vi "File Control Time Check.vi"() -> ()   [LabVIEW 2015]
uses:
  <vilib>/Utility/sysdir.llb/System Directory Type.ctl
panel:
  out "x*y":dbl
  out "Data Logging Path":path
  in  "Log no":string="1" caption="No."
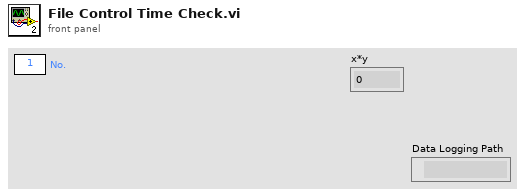
[diagram p1: front panel]
types:
  T1 = enum16{"open", "replace", "create", "open or create", "replace or create", "replace or create with confirmation"}
  T2 = typedef "System Directory Type.ctl" = i32
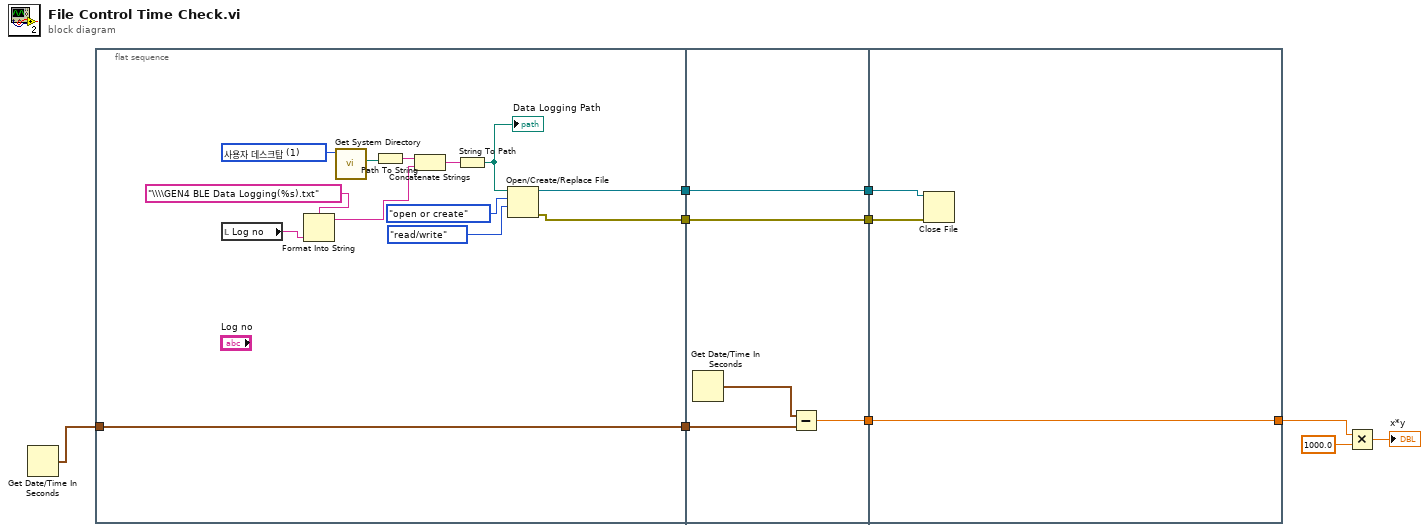
[diagram p0: block diagram]
diagram:
  n1 = Get Date/Time In Seconds() -> (seconds since 1Jan1904=w10:timestamp)
  n2 = flat-sequence {
    tunnel: w10 -> [w13]
    tunnel: [w13] -> w9
    tunnel: [w12] -> w8
    tunnel: [w11] -> w5
    tunnel: w9 -> [w27]
    tunnel: w8 -> [w26]
    tunnel: [w26] -> w7
    tunnel: [w25] -> w6
    tunnel: w5 -> [w25]
    tunnel: [w24] -> w4
    tunnel: w7 -> [w31]
    tunnel: w6 -> [w30]
    tunnel: [w29] -> w3
    tunnel: w4 -> [w29]
    frame #0 {
      w23 = T2 1 items=["사용자 홈"=0, "사용자 데스크탑"=1, "사용자 문서"=2, "사용자 어플리케이션 데이터"=3, "사용자 환경"=4, "사용자 임시"=5, "퍼블릭 문서"=6, "퍼블릭 어플리케이션 데이터"=7, "퍼블릭 환경"=8, "퍼블릭 캐시"=13, "시스템 코어 라이브러리"=9, "시스템 설치된 라이브러리"=10, "어플리케이션 파일"=11, "부팅 볼륨 루트"=12] ("system directory type")
      n3 = local read "Log no"() -> (w14:string)
      n4 = Format Into String(format string="\\\\GEN4 BLE Data Logging(%s).txt" ("문자열"), w14) -> (resulting string=w15:string)  [unwired: 2 in, 1 out]
      n5 = call <vilib>:"Get System Directory.vi"("system directory type"=w23) -> ("system directory"=w22:path)  [unwired: 10 in]
      n6 = Path To String(path=w22) -> (string=w21:string)
      n7 = Concatenate Strings(w21, w15) -> (w20:string)
      n8 = String To Path(string=w20) -> (path=w19:path)
      "Data Logging Path" <- w19
      n9 = Open/Create/Replace File(file path (use dialog)=w19, operation (0:open)=T1."open or create" ("동작(0:open)"), access (0:read/write)=enum16{"read/write", "read-only", "write-only"}."read/write" ("접근(0:읽기/쓰기)")) -> (refnum out=w12:refnum<file>, error out=w11:errorcluster)  [unwired: 3 in, 1 out]
    }
    frame #1 {
      n10 = Get Date/Time In Seconds() -> (seconds since 1Jan1904=w28:timestamp)
      n11 = Subtract(x=w28, y=w27) -> (x-y=w24:dbl)
    }
    frame #2 {
      n12 = Close File(refnum=w31, error in=w30) -> ()  [unwired: 2 out]
    }
  }
  n13 = Multiply(x=w3, y=1000.0) -> (x*y=→"x*y":dbl)
